vi "premat.vi"(1 "Eq2":dbl, 2 "Eq1":dbl) -> (0 "Premat":dbl[][](array[numeric]) format="%.11g")   [LabVIEW 2019]
panel:
  out "C":dbl format="%#_12g"
  out "B":dbl format="%#_12g"
  out "A":dbl format="%_12g"
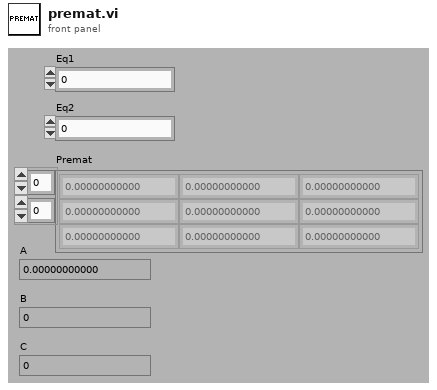
[diagram p1: front panel]
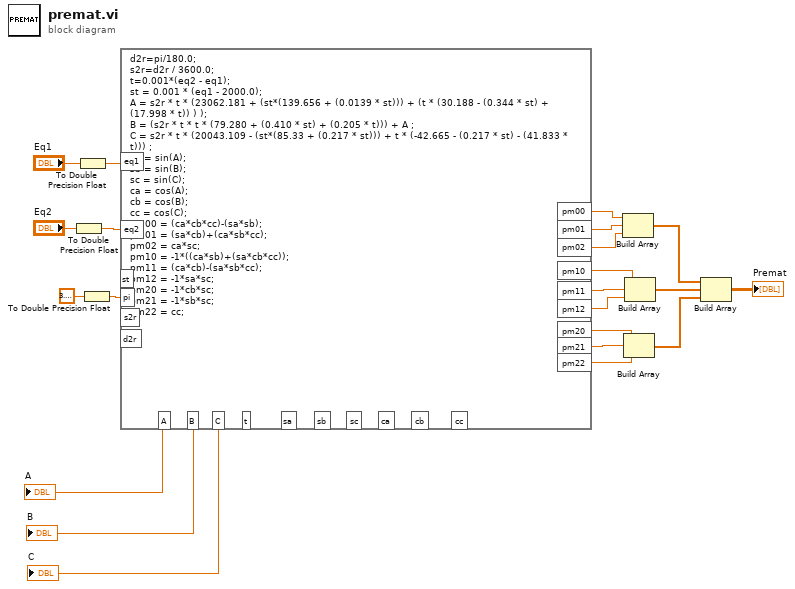
[diagram p0: block diagram]
diagram:
  n1 = To Double Precision Float(number="Eq2") -> (double precision float=w12:dbl)
  n2 = To Double Precision Float(number="Eq1") -> (double precision float=w13:dbl)
  n3 = To Double Precision Float(number=3.141592653589793) -> (double precision float=w1:dbl)
  n4 = formula code="d2r=pi/180.0;\ns2r=d2r / 3600.0;\nt=0.001*(eq2 - eq1);\nst = 0.001 * (eq1 - 2000.0);\nA = s2r * t * (23062.181 + (st*(139.656 + (0.0139 * st))) + (t * (30.188 - (0.344 * st) + (17.998 * t)) ) );\nB = (s2r * t * t * (79.280 + (0.410 * st) + (0.205 * t))) + A ;\nC = s2r * t * (20043.109 - (st*(85.33 + (0.217 * st))) + t * (-42.665 - (0.217 * st) - (41.833 * t))) ;\nsa = sin(A);\nsb = sin(B);\nsc = sin(C);\nca = cos(A);\ncb = cos(B);\ncc = cos(C);\npm00 = (ca*cb*cc)-(sa*sb);\npm01 = (sa*cb)+(ca*sb*cc);\npm02 = ca*sc;\npm10 = -1*((ca*sb)+(sa*cb*cc));\npm11 = (ca*cb)-(sa*sb*cc);\npm12 = -1*sa*sc;\npm20 = -1*cb*sc;\npm21 = -1*sb*sc;\npm22 = cc;"("pi"=w1, "eq1"=w13, "eq2"=w12) -> ("A"=→"A":dbl, "B"=→"B":dbl, "C"=→"C":dbl, "pm00"=w14:dbl, "pm01"=w15:dbl, "pm02"=w16:dbl, "pm10"=w11:dbl, "pm11"=w10:dbl, "pm12"=w9:dbl, "pm20"=w8:dbl, "pm21"=w7:dbl, "pm22"=w6:dbl)  [unwired: 10 out]
  n5 = Build Array(w14, w15, w16) -> (w5:dbl[])
  n6 = Build Array(w8, w7, w6) -> (w3:dbl[])
  n7 = Build Array(w11, w10, w9) -> (w4:dbl[])
  n8 = Build Array(w5, w4, w3) -> (→"Premat":dbl[][])
